vi "main.vi"() -> ()   [LabVIEW 2014]
uses:
  libraryGcode/ControlGlobal/stateModeDevice.ctl
  libraryGcode/control/stateBoardFirmware.ctl
  libraryGcode/control/Queue/QueueCMDandPOS.ctl
  libraryGcode/control/Queue/TypeDataPOS.ctl
  libraryGcode/control/stateCmdUpdatePara.ctl
  C/Users/annha/Desktop/Inverse Kinematic - demo/controls/Robot_definition.ctl
  LIN3D/Robot_testing_instructions.ctl
  libraryGcode/control/TypeFirmwareControl.ctl
  libraryGcode/ClassStringGcode/XuLyDataDisplay.lvclass
  <vilib>/Platform/TimedLoop/XDataNode/timing_clust.ctl
  <vilib>/Platform/TimedLoop/XDataNode/nitl_modes.ctl
  <vilib>/Platform/TimedLoop/XDataNode/wakeup.ctl
  libraryGcode/ClassParameter/stateLoop_View.ctl
  libraryGcode/ClassStringGcode/SelectMcode.ctl
  libraryGcode/ClassStringGcode/SelectGcode.ctl
  libraryGcode/variableGlobal/StartAutoandGcode.vi
  <vilib>/Platform/TimedLoop/XDataNode/XDataNode.xnode
  libraryGcode/LibraryGcode.lvlib
  <vilib>/Platform/TimedLoop/XDataNode/XDNodeRunTimeDep.lvlib
  <vilib>/picture/3D Picture Control/NI_3D Picture Control.lvlib
  libraryGcode/ClassParameter/ParameterConf.lvclass
panel:
  out "degrees":cluster{"A":dbl, "B":dbl}
  out "error out 2":errorcluster
  out "error out":errorcluster
  out "data GET":string="w\n"
  out "POS":cluster{"X":dbl, "Y":dbl, "Z":dbl}
  out "STATE BOARD":T1=enum."Waiting"
  out "statusMode":T2=enum."Menu"
  in  "SwitchMode":bool
  in  "Exit Program":bool=TRUE
  in  "Tab Control":enum32{"Setting", "Auto", "Config", ""}(tab)
  out "G2-G3 PARA":cluster{"X":dbl, "Y":dbl, "I":dbl, "J":dbl}
  in  "Send Gcode manual":T3
  in  "BUTTON CONTROL GCODE FILE":T4={"FILE"={"AddFile_ButtonSaveFile"=FALSE, "AddFile_ButtonDeleteLastLine"=FALSE, "AddFile_ButtonDeleteAll"=FALSE}, "MOTION"={"AddFile_ButtonGoHome"=TRUE, "AddFile_ButtonAddG1"=FALSE, "AddFile_ButtonAddG0"=FALSE}}
  in  "BUTTON CONTROL MANUAL":T5
  in  "PARA":cluster{"STEP":i16, "FEEDRATE":dbl}={"STEP"=10, "FEEDRATE"=500.0} {"FEEDRATE" min=0.0 max=10000.0 step=50.0; "STEP" min=0 max=90 step=2 format="%-1.0f"}
  in  "CONTROL PWM":T6={"SPIN"={"PWM"=55.0, "Control_buttonSpindle"=FALSE, "ButtonSPINDLE_ADD_FILE"=FALSE}, "FAN 1"={"Control_ButtonFan1"=FALSE, "PWM"=255.0, "AddFile_ButtonFan1"=FALSE}, "FAN 2"={"PWM"=0.0, "Control_ButtonFan2"=FALSE, "AddFile_ButtonFan2"=FALSE}, "FAN 3"={"PWM"=0.0, "Control_ButtonFan3"=FALSE, "AddFile_ButtonFan3"=FALSE}, "WAIT PIN"={"PIN INPUT"=55.0, "Control_ButtonWaitPin"=FALSE, "AddFile_ButtonWaitPin"=FALSE}, "SOLENOID"={"Control_ButtonSolenoid"=FALSE, "AddFile_ButtonSolenoid"=FALSE}} {"WAIT PIN"."PIN INPUT" min=55.0 max=58.0 step=1.0; "FAN 3"."PWM" min=0.0 max=255.0 step=5.0; "FAN 2"."PWM" min=0.0 max=255.0 step=5.0; "FAN 1"."PWM" min=0.0 max=255.0 step=10.0; "SPIN"."PWM" min=0.0 max=255.0 step=1.0}
  in  "Link Save File":path
  out "GCODE ADD":string="\r"
  in  "File to Cut":path
  in  "Start Auto":bool
  out "G-Code Array 2":string[](array[string])=["Loi khong ket noChua Chon File"]
  in  "RESET ERROR":bool
  in  "MAX FEEDRATE":T7={"DATA"={"X"=4000.0, "Y"=4000.0, "Z"=4000.0}, "Config_SetFeedrate"=FALSE}
  in  "MAX ACCEL":T8={"DATA"={"X"=5000.0, "Y"=5000.0, "Z"=500.0}, "Config_SetMaxACCEL"=FALSE}
  in  "STEPSIZE":T9={"DATA"={"X"=88.89, "Y"=88.89, "Z"=2133.33}, "Config_SetStepSize"=FALSE}
  in  "M204 Start AcceL":T10={"Config_SetSTARTACCEL"=FALSE, "data"={"P"=88.89, "R"=88.89, "T"=2133.33}}
  in  "Move":cluster{"X":dbl, "Y":dbl, "OK Button":bool}
  in  "Config_SaveEEPROM":bool
  out "output cluster 2":cluster{"angle 1":dbl, "angle 2":dbl, i32}
  out "3D Picture":refnum<vi>(3d-picture)
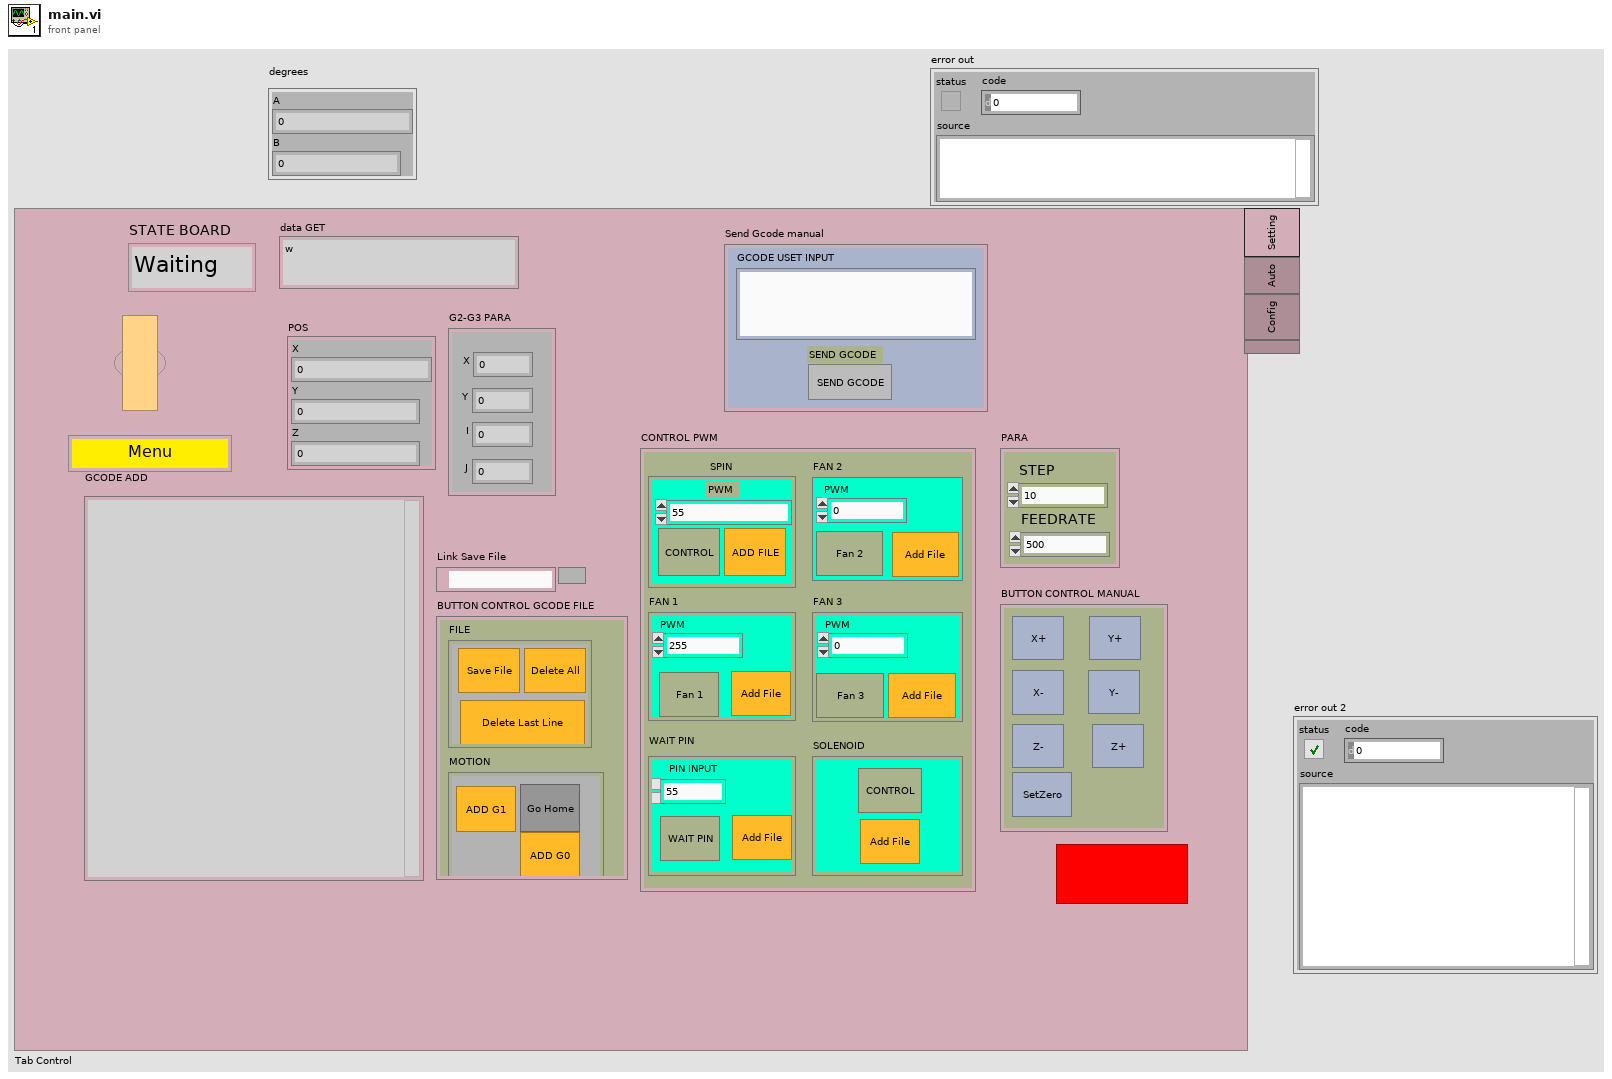
[diagram p1: front panel]
types:
  T1 = typedef "LibraryGcode.lvlib/stateBoardFirmware.ctl" = enum16{"Running", "Waiting", "Pos", "IDLE"}
  T2 = typedef "stateModeDevice.ctl" = enum16{"Auto", "Menu", "WaitAutoFinish", "Config", "initAuto"}
  T3 = cluster{"GCODE USET INPUT":string, "SEND GCODE":bool}
  T4 = cluster{"FILE":cluster{"AddFile_ButtonSaveFile":bool, "AddFile_ButtonDeleteLastLine":bool, "AddFile_ButtonDeleteAll":bool}, "MOTION":cluster{"AddFile_ButtonGoHome":bool, "AddFile_ButtonAddG1":bool, "AddFile_ButtonAddG0":bool}}
  T5 = cluster{"Control_ButtonX+":bool, "Control_ButtonX-":bool, "Control_ButtonY+":bool, "Control_ButtonY-":bool, "Control_ButtonZ+":bool, "Control_ButtonZ-":bool, "Control_ButtonSetZero":bool}
  T6 = cluster{"SPIN":cluster{"PWM":dbl, "Control_buttonSpindle":bool, "ButtonSPINDLE_ADD_FILE":bool}, "FAN 1":cluster{"Control_ButtonFan1":bool, "PWM":dbl, "AddFile_ButtonFan1":bool}, "FAN 2":cluster{"PWM":dbl, "Control_ButtonFan2":bool, "AddFile_ButtonFan2":bool}, "FAN 3":cluster{"PWM":dbl, "Control_ButtonFan3":bool, "AddFile_ButtonFan3":bool}, "WAIT PIN":cluster{"PIN INPUT":dbl, "Control_ButtonWaitPin":bool, "AddFile_ButtonWaitPin":bool}, "SOLENOID":cluster{"Control_ButtonSolenoid":bool, "AddFile_ButtonSolenoid":bool}}
  T7 = cluster{"DATA":cluster{"X":dbl, "Y":dbl, "Z":dbl}, "Config_SetFeedrate":bool}
  T8 = cluster{"DATA":cluster{"X":dbl, "Y":dbl, "Z":dbl}, "Config_SetMaxACCEL":bool}
  T9 = cluster{"DATA":cluster{"X":dbl, "Y":dbl, "Z":dbl}, "Config_SetStepSize":bool}
  T10 = cluster{"Config_SetSTARTACCEL":bool, "data":cluster{"P":dbl, "R":dbl, "T":dbl}}
  T11 = typedef "Robot_testing_instructions.ctl" = enum16{"idle", "Draw Robot", "Init 1 - Application", "Quit", "Close", "Error Handling", "Calculates"}
  T12 = typedef "Robot_definition.ctl" = cluster{"L2":sgl, "L3":sgl, "L1":sgl, "Base":sgl, "X0":sgl, "Z0":sgl}
  T13 = cluster{"Scene ref":refnum<vi>, "Arm 1 ref":refnum<vi>, "Arm 2 ref":refnum<vi>, "Arm 1 offset":cluster{"X":sgl, "Y":sgl, "Z":sgl}[], "Arm 2 offset":cluster{"X":sgl, "Y":sgl, "Z":sgl}[], "sand box":refnum<vi>, "Status":string, "A1":dbl, "A2":dbl, "Robot Definition":T12}
  T14 = typedef "LibraryGcode.lvlib/stateCmdUpdatePara.ctl" = enum16{"updatePos", "UpdateConfigAccel", "UpdateConfigFeed", "UpdateConfigUnit", "UpdateConfigStartAccel", "NoUpdate"}
  T15 = cluster{"Command":T14, "POS":cluster{"X":dbl, "Y":dbl, "Z":dbl}, "DEGREES":cluster{"X":dbl, "Y":dbl}}
  T16 = typedef "LibraryGcode.lvlib/QueueCMDandPOS.ctl" = cluster{"Serial Data Gcode":refnum<queue>, "cmdUpdateDisplay":refnum<queue>}
  T17 = typedef "LibraryGcode.lvlib/TypeFirmwareControl.ctl" = enum16{"ScaraMarlin", "CncMarlin", "Mk4Due"}
  T18 = typedef "XDNodeRunTimeDep.lvlib/timing_clust.ctl" = cluster{"Expected End [f-1]":u64, "Actual End [f-1]":u64, "Finished Late? [f-1]":bool, "Expected End [i-1]":u64, "Actual End [i-1]":u64, "Finished Late? [i-1]":bool, "Expected Start [i]":u64, "Actual Start [i]":u64, "Expected Start [f]":u64, "Actual Start [f]":u64, "Source Name":string, "Structure Name":string, "Period":i64, "Deadline":i64, "Offset":i64, "Start":i64, "Priority":i32, "Timeout":i32, "Mode":T19, "Wakeup Reason":T20, "Error":errorcluster, "Source Type":string, "Secondary Source Type":string, "Global End Time":u64, "Global Start Time":u64, "Frame Duration":u64, "Iteration Duration":u64, "Assigned CPU":i32, "I/O Scan Engine Mode":u32}
  T19 = typedef "XDNodeRunTimeDep.lvlib/nitl_modes.ctl" = enum32{"No Change", "Process missed periods, maintain original phase", "Discard missed periods, maintain original phase", "Process missed periods, ignore original phase", "Discard missed periods, ignore original phase"}
  T20 = typedef "XDNodeRunTimeDep.lvlib/wakeup.ctl" = enum32{"Normal", "Aborted", "Asynchronous wakeup", "Timing source error", "Timed loop error", "Timeout"}
  T21 = typedef "LibraryGcode.lvlib/XuLyDataDisplay.lvclass/SelectMcode.ctl" = enum16{"M204_SetStartingAcceleration", "M503_ReportSetting", "M500_SaveEprom", "M114_GetPosition", "M92_SetAxisStepPerUnit", "M17_EnableStep", "M18_DisableStep", "M80_PowerOn", "M81_PowerOff", "M112_EMGStop", "M118_SerialPrint", "M226_WaitforPinState", "M400_WaitFinishMove", "M203_SetMaxFeedRate", "M201_SetMaxACCEL", "M380_381_SetSoleNoid_On_Off", "M42_InitPin", "M42_PinControl", "M106_SetFan1", "M106_SetFan2", "M106_SetFan3", "M3_SetSpindle", "M5_OffSpindle", "M999_RestartStop"}
  T22 = typedef "LibraryGcode.lvlib/ParameterConf.lvclass/stateLoop_View.ctl" = enum16{"Running", "writeGlobal", "schedules500ms", "init", "End"}
  T23 = enum16{"Fan1", "Fan2", "Fan3", "PARA", "POS_DEGREE", "Solenoid", "Spindle", "TypeFirmware", "WaitPin", "MaxAcel", "MaxFeedrate", "MaxSize", "MaxStartAccel"}
  T24 = typedef "LibraryGcode.lvlib/XuLyDataDisplay.lvclass/SelectGcode.ctl" = enum16{"G0LinearMove", "G1XY", "G1LinearMove", "G2Arc", "G4Dwell", "G20InchUnit", "G21MilliUnit", "G28AutoHome", "G92SetPosition", "G90", "G91RelativePos", "JogX+", "JogX-", "JogY+", "JogY-", "JogZ+", "JogZ-", "sendGcodeString"}
  T25 = cluster{"SPIN":dbl, "FAN2":dbl, "FAN1":dbl, "FAN3":dbl, "WAIT PIN ":dbl}
  T26 = cluster{"PWM":dbl, "TypeFirmware":T17, "XYZ":cluster{"X":dbl, "Y":dbl, "Z":dbl}, "PARA":cluster{"STEP":i16, "FEEDRATE":dbl}, "DEGREES":cluster{"X":dbl, "Y":dbl}, "Solenoid":bool, "StartAccel":cluster{"P":dbl, "R":dbl, "T":dbl}}
  T27 = typedef "Robot_creation_loop_data.ctl" = cluster{"Robot Definition":T12, "Dispenser ref":refnum<vi>, "Arm 2 ref":refnum<vi>, "Arm 1 ref":refnum<vi>, "Base ref":refnum<vi>, "Scene ref":refnum<vi>, "Sand box ref":refnum<vi>, "Arm 1 Offset":cluster{"X":sgl, "Y":sgl, "Z":sgl}[], "Arm 2 Offset":cluster{"X":sgl, "Y":sgl, "Z":sgl}[], "Width":sgl}
  T28 = cluster{"error out":errorcluster, "error IO 2":errorcluster}
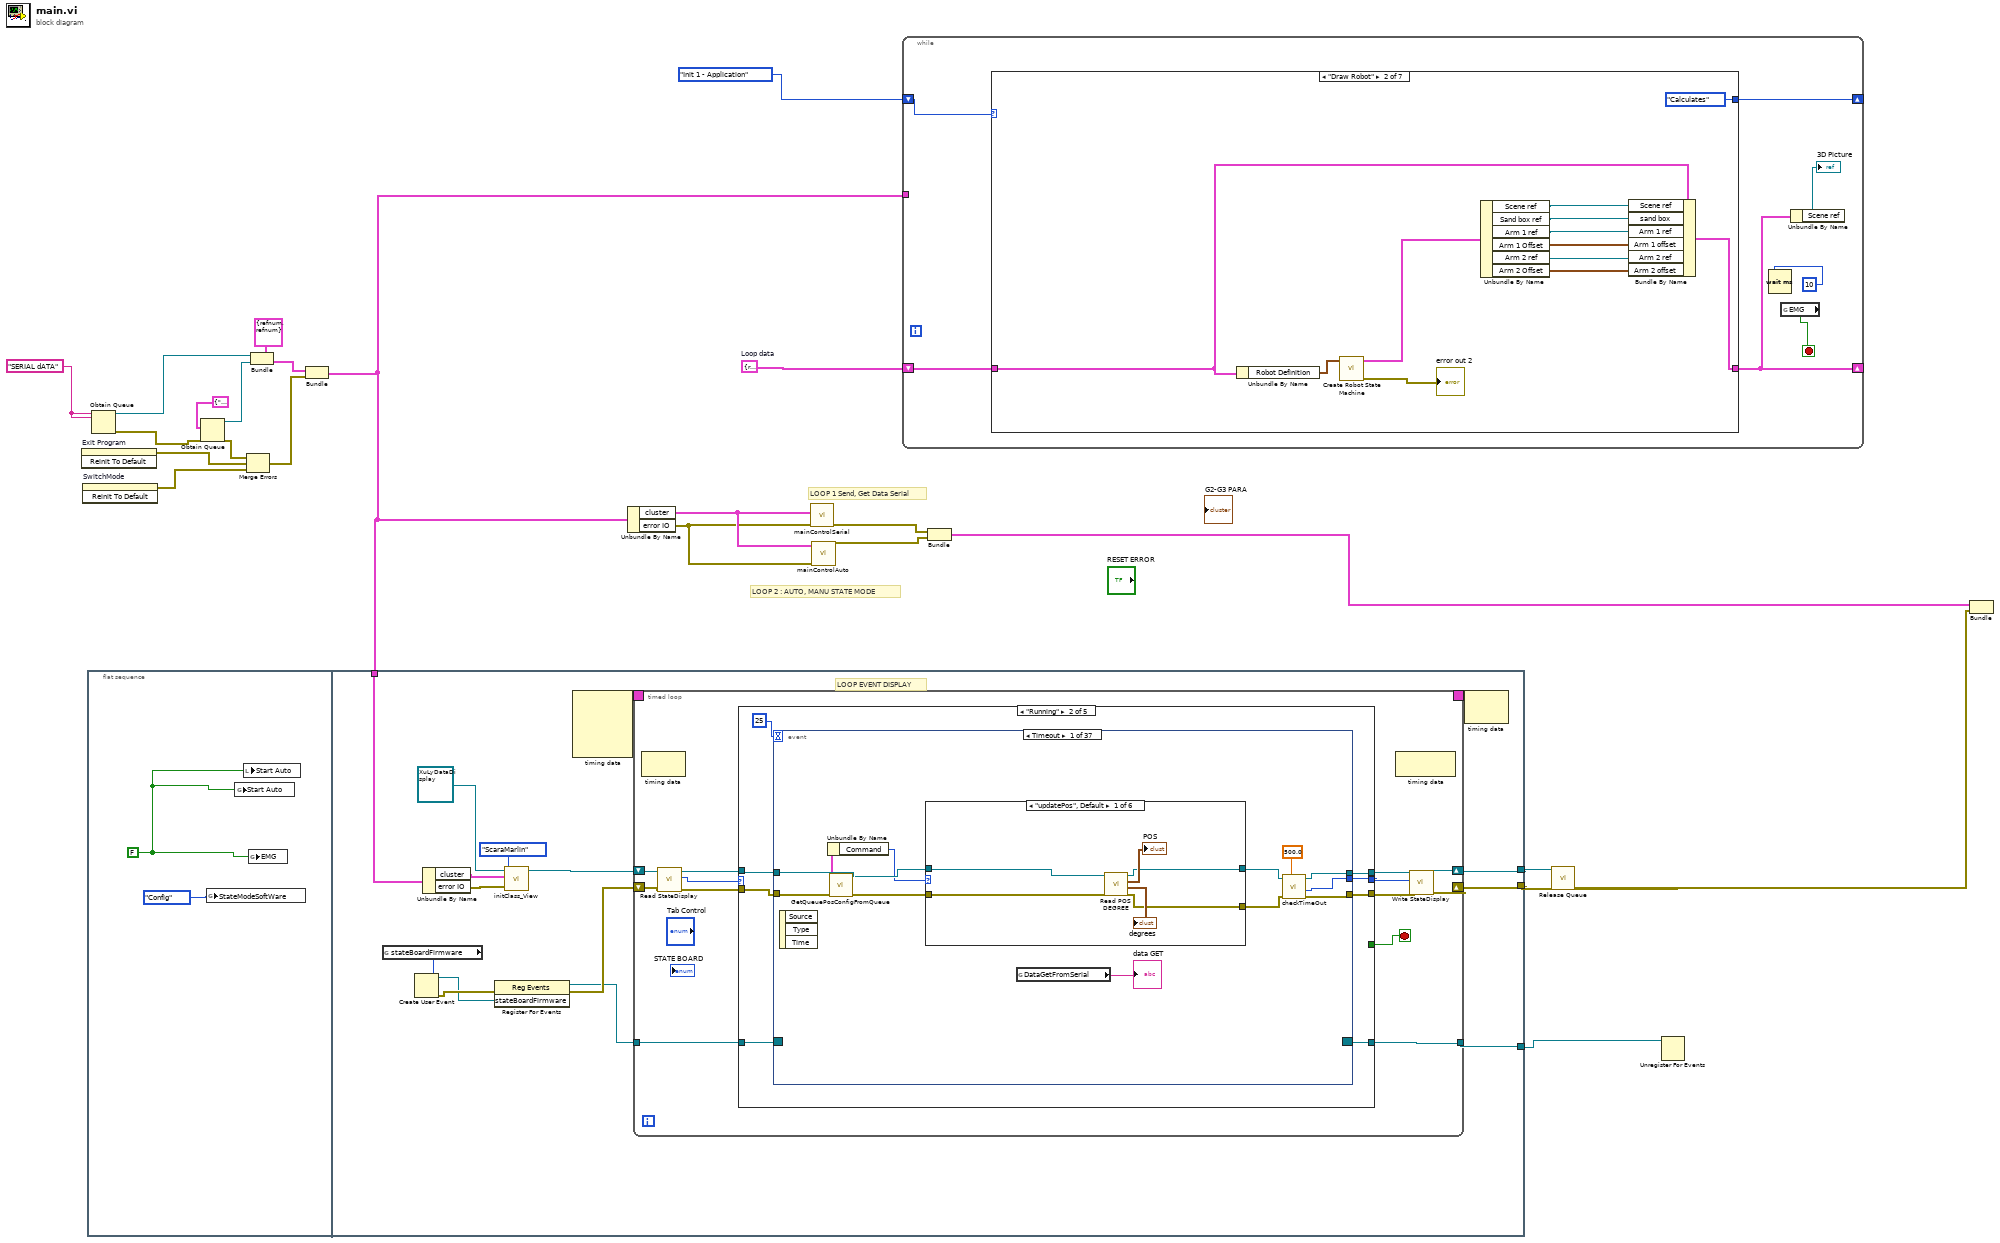
[diagram p0: block diagram]
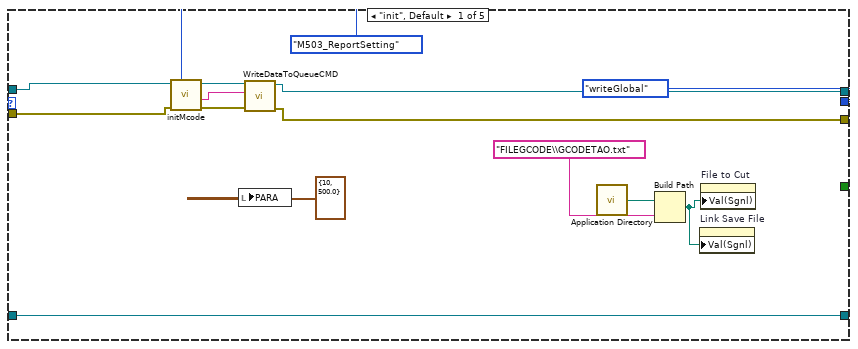
[diagram p2: hidden frame]
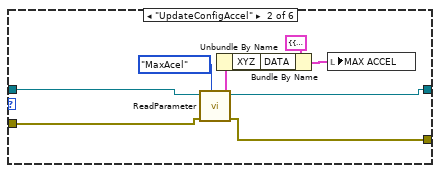
[diagram p3: hidden frame]
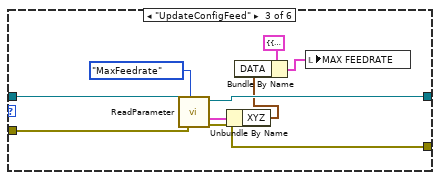
[diagram p4: hidden frame]
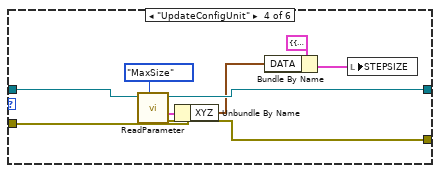
[diagram p5: hidden frame]
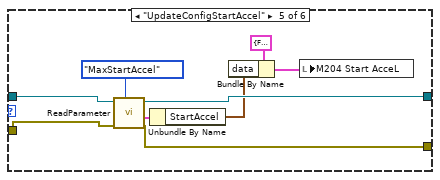
[diagram p6: hidden frame]
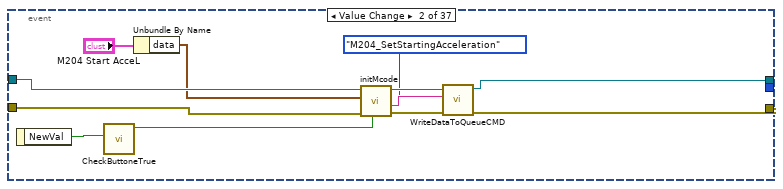
[diagram p8: hidden frame]
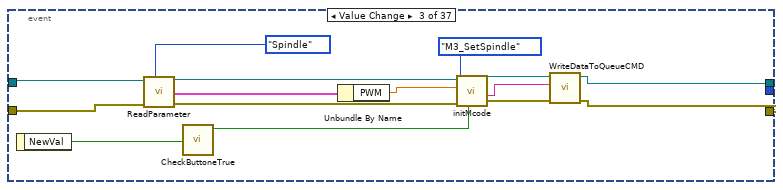
[diagram p9: hidden frame]
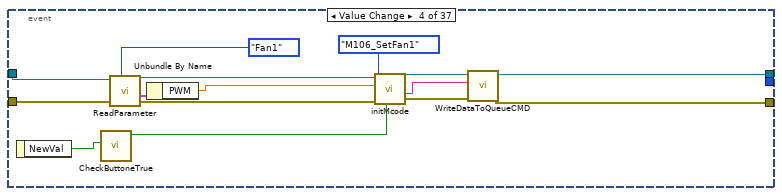
[diagram p10: hidden frame]
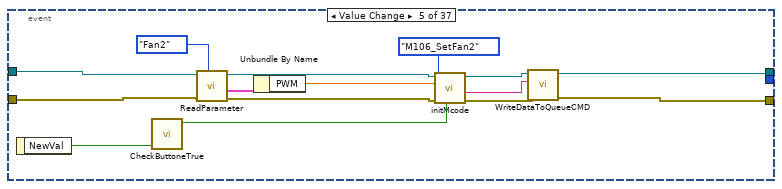
[diagram p11: hidden frame]
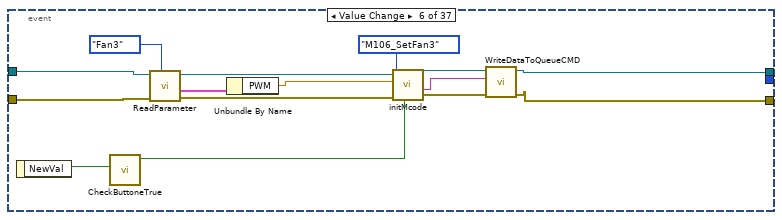
[diagram p12: hidden frame]
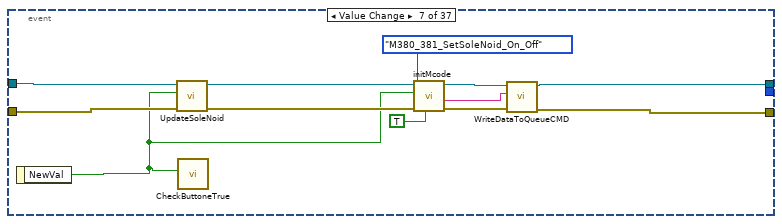
[diagram p13: hidden frame]
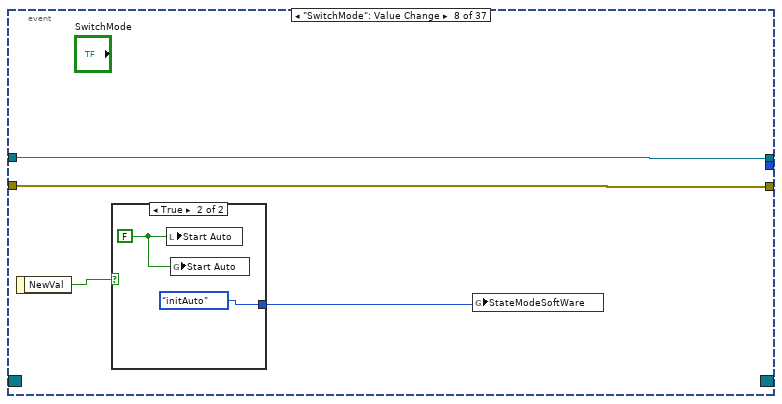
[diagram p14: hidden frame]
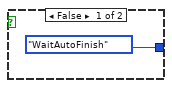
[diagram p15: hidden frame]
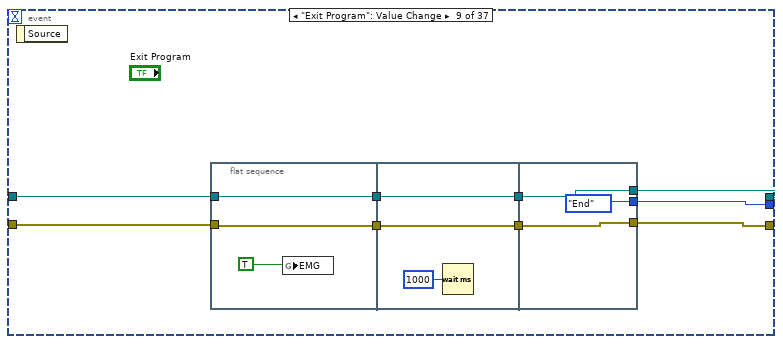
[diagram p16: hidden frame]
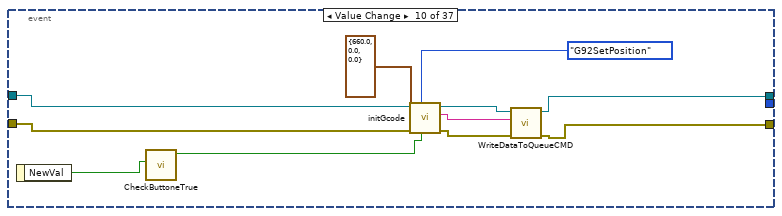
[diagram p17: hidden frame]
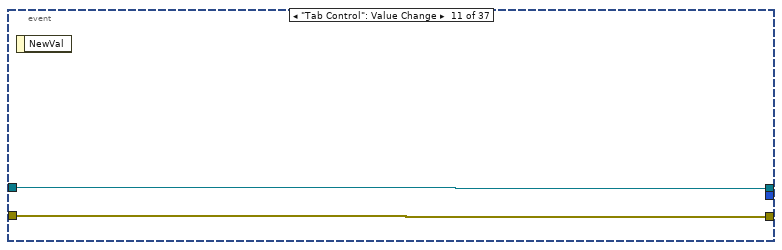
[diagram p18: hidden frame]
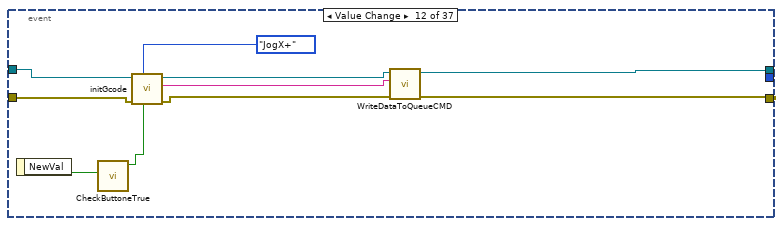
[diagram p19: hidden frame]
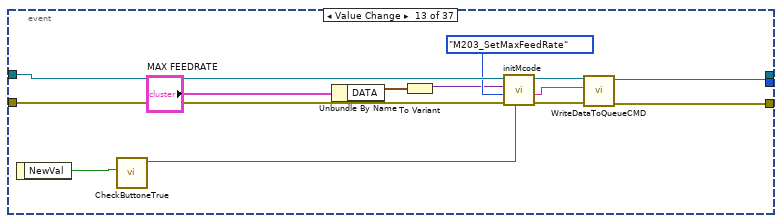
[diagram p20: hidden frame]
diagram:
  w9 = T13 {"Scene ref"=refnum, "Arm 1 ref"=refnum, "Arm 2 ref"=refnum, "Arm 1 offset"=[], "Arm 2 offset"=[], "sand box"=refnum, "Status"="", "A1"=43.0, "A2"=23.0, "Robot Definition"={"L2"=0.0, "L3"=0.0, "L1"=0.0, "Base"=0.0, "X0"=0.0, "Z0"=0.0}}  # Loop data
  w23 = "SERIAL dATA" ("name (unnamed)")
  # "LOOP 2 : AUTO, MANU STATE MODE"
  # "LOOP 1 Send, Get Data Serial"
  n1 = invoke on="Exit Program" class="Bool" method="Reinit To Default"() -> (error out=w21:errorcluster)  [unwired: 3 in, 2 out]
  n2 = invoke on="SwitchMode" class="Bool (strict)" method="Reinit To Default"() -> (error out=w22:errorcluster)  [unwired: 3 in, 2 out]
  n3 = flat-sequence {
    tunnel: [w41] -> w3
    tunnel: w11 -> [w40]
    tunnel: [w37] -> w4
    tunnel: [w27] -> w1
    frame #0 {
      w25 = FALSE ("Start Auto")
      n4 = global write "StartAutoandGcode.vi" "StateModeSoftWare"(stateModeDevice."Config" ("Enum")) -> ()
      n5 = global write "StartAutoandGcode.vi" "Start Auto"(w25) -> ()
      n6 = local write "Start Auto"(w25) -> ()
      n7 = global write "StartAutoandGcode.vi" "EMG"(w25) -> ()
    }
    frame #1 {
      # "LOOP EVENT DISPLAY"
      n8 = global read "StartAutoandGcode.vi" "stateBoardFirmware"() -> (w29:T1)
      n9 = Create User Event(user event datatype=w29) -> (user event=w28:refnum<user-event>, error out=w31:errorcluster)  [unwired: 1 in]
      n10 = Unbundle By Name(w40) -> ("cluster"=w36:T16, "error IO"=w26:errorcluster)
      n11 = register-events(error in=w31, w28) -> (reference out=w30:refnum<event-registration>, error out=w32:errorcluster)  [unwired: 1 in]
      n12 = call-dynamic "initClass_View.vi"("error in (no error)"=w26, "TypeFirmware"=TypeFirmwareControl."ScaraMarlin", "Queue Process"=w36, "XuLyDataDisplay in"=refnum<class "XuLyDataDisplay.lvclass"> refnum) -> ("XuLyDataDisplay out"=w34:refnum<class "XuLyDataDisplay.lvclass">)  [unwired: 6 in, 1 out]
      n13 = node-c288() -> (w39:T18)  [unwired: 4 in]
      n14 = timed-loop {
        timing: w39 -> [_]
        timing-out: [_] -> w38
        shift-right: [w49] -> w37
        shift-left: w34 -> [w53]
        shift-right: [w48] -> w41
        shift-left: w32 -> [w51]
        tunnel: w30 -> [w43]
        tunnel: [w42] -> w27
        stop <- w54 stop-if-true
        n15 = node-c288() -> ()  [unwired: 1 in, 1 out]
        n16 = call-dynamic "Read StateDisplay.vi"("error in (no error)"=w51, "ParameterConf in"=w53) -> ("error out"=w50:errorcluster, "StateDisplay"=w46:T22, "ParameterConf out"=w52:refnum<class "XuLyDataDisplay.lvclass">)  [unwired: 7 in]
        n17 = case shown="\"Running\"" w46 {
          tunnel: w50 -> [w61 w71 w542 w554 w571]
          tunnel: [_ _ TRUE _ _] -> w54
          tunnel: [w60 w75 w542 w552 w568] -> w47
          tunnel: w52 -> [w65 w77 w541 w555 w572]
          tunnel: [w62 w73 w541 w553 w569] -> w44
          tunnel: [stateLoop_View."writeGlobal" ("StateDisplay") w76 stateLoop_View."init" ("StateDisplay") stateLoop_View."schedules500ms" ("StateDisplay") stateLoop_View."Running" ("StateDisplay")] -> w45
          tunnel: w43 -> [w57 w74 w539 w544 w566]
          tunnel: [w57 w72 w539 w544 w566] -> w42
          frame "init", Default {
            n18 = call-dynamic "initMcode.vi"("error in (no error)"=w61, "mCode"=SelectMcode."M503_ReportSetting", "XuLyDataDisplay in"=w65) -> ("error out"=w59:errorcluster, "McodeOut"=w63:string, "XuLyDataDisplay out"=w64:refnum<class "XuLyDataDisplay.lvclass">)  [unwired: 6 in]
            n19 = local write "PARA"(cluster{"STEP":i16, "FEEDRATE":dbl} {"STEP"=10, "FEEDRATE"=500.0} ("PARA")) -> ()
            n20 = call-dynamic "WriteDataToQueueCMD.vi"("error in (no error)"=w59, "DataIn"=w63, "ParameterConf in"=w64) -> ("error out"=w60:errorcluster, "ParameterConf out"=w62:refnum<class "XuLyDataDisplay.lvclass">)  [unwired: 7 in]
            n21 = call <vilib>:"Application Directory.vi"() -> ("Application Directory"=w68:path)
            n22 = Build Path(base path=w68, name or relative path="FILEGCODE\\GCODETAO.txt") -> (appended path=w70:path)
            n23 = property on="Link Save File" class="Path"("Val(Sgnl)"=w70) -> ()  [unwired: 2 in, 2 out]
            n24 = property on="File to Cut" class="Path"("Val(Sgnl)"=w70) -> ()  [unwired: 2 in, 2 out]
          }
          frame "Running" {
            n25 = event shown="[0] Timeout" {
              selector: w74 -> [_ _ _ _ _ _ _ _ _ _ _ _ _ _ _ _ _ _ _ _ _ _ _ _ _ _ _ _ _ _ _ _ _ w498 _ _ _]
              dyn-events: [_ _ _ _ _ _ _ _ _ _ _ _ _ _ _ _ _ _ _ _ _ _ _ _ _ _ _ _ _ _ _ _ _ w498 _ _ _] -> w72
              timeout: 25 -> [_ _ _ _ _ _ _ _ _ _ _ _ _ _ _ _ _ _ _ _ _ _ _ _ _ _ _ _ _ _ _ _ _ _ _ _ _]
              tunnel: w71 -> [w90 w140 w160 w175 w190 w206 w218 w223 w229 w252 w257 w262 w274 w290 w299 w313 w326 w332 w344 w357 w363 w382 w397 w408 w425 w440 w446 w450 w452 w461 w473 w483 w495 w506 w516 w522 w532]
              tunnel: [w82 w143 w151 w171 w184 w200 w212 w223 w228 w247 w257 w260 w276 w285 w301 w310 w321 w332 w336 w357 w362 w369 w385 w400 w415 w428 w443 w450 w453 w464 w467 w484 w493 w502 w509 w519 w531] -> w75
              tunnel: w77 -> [w91 w146 w161 w176 w191 w205 w219 w222 w232 w253 w256 w263 w278 w291 w304 w314 w328 w331 w345 w358 w364 w383 w398 w409 w426 w441 w447 w449 w455 w463 w474 w486 w496 w507 w517 w523 w533]
              tunnel: [w83 w144 w152 w172 w185 w201 w215 w222 w235 w248 w256 w258 w275 w286 w302 w311 w319 w331 w335 w358 w359 w370 w386 w401 w416 w429 w444 w449 w451 w456 w468 w485 w494 w503 w510 w520 w529] -> w73
              tunnel: [w80 _ _ _ _ _ _ _ w227 _ _ _ _ _ _ _ _ _ _ stateLoop_View."writeGlobal" ("StateDisplay") _ _ _ _ _ _ _ _ _ _ _ _ _ _ _ _ _] -> w76
              event Timeout {
                n26 = event-data() -> ()  [unwired: 1 in, 3 out]
                n27 = call-dynamic "GetQueuePosConfigFromQueue.vi"("error in (no error)"=w90, "ParameterConf in"=w91) -> ("error out"=w87:errorcluster, "element"=w89:T15, "ParameterConf out"=w88:refnum<class "XuLyDataDisplay.lvclass">)  [unwired: 7 in]
                n28 = Unbundle By Name(w89) -> ("Command"=w79:T14)
                n29 = case shown="\"updatePos\", Default" w79 {
                  tunnel: [w93 w106 w113 w123 w132 w135] -> w85
                  tunnel: w88 -> [w95 w105 w115 w116 w128 w135]
                  tunnel: [w92 w103 w112 w122 w131 w134] -> w84
                  tunnel: w87 -> [w94 w104 w114 w124 w133 w134]
                  frame "updatePos", Default {
                    n30 = call-dynamic "Read POS DEGREE.vi"("error in (no error)"=w94, "ParameterConf in"=w95) -> ("error out"=w92:errorcluster, "DEGREES"=→"degrees":cluster{"X":dbl, "Y":dbl}, "POS"=→"POS":cluster{"X":dbl, "Y":dbl, "Z":dbl}, "ParameterConf out"=w93:refnum<class "XuLyDataDisplay.lvclass">)  [unwired: 6 in]
                  }
                  frame "UpdateConfigAccel" {
                    n31 = call-dynamic "ReadParameter.vi"("ParameterConf in"=w105, "error in (no error)"=w104, "Parameter"=T23."MaxAcel") -> ("ParameterConf out"=w106:refnum<class "XuLyDataDisplay.lvclass">, "DataOutClust"=w99:T26, "error out"=w103:errorcluster)  [unwired: 4 in, 1 out]
                    n32 = Unbundle By Name(w99) -> ("XYZ"=w98:cluster{"X":dbl, "Y":dbl, "Z":dbl})
                    n33 = Bundle By Name(cluster=T8 {"DATA"={"X"=355.0, "Y"=355.0, "Z"=2133.0}, "Config_SetMaxACCEL"=FALSE} ("MAX ACCEL"), "DATA"=w98) -> (w101:T8)
                    n34 = local write "MAX ACCEL"(w101) -> ()
                  }
                  frame "UpdateConfigFeed" {
                    n35 = call-dynamic "ReadParameter.vi"("ParameterConf in"=w115, "error in (no error)"=w114, "Parameter"=T23."MaxFeedrate") -> ("ParameterConf out"=w113:refnum<class "XuLyDataDisplay.lvclass">, "DataOutClust"=w108:T26, "error out"=w112:errorcluster)  [unwired: 4 in, 1 out]
                    n36 = Unbundle By Name(w108) -> ("XYZ"=w107:cluster{"X":dbl, "Y":dbl, "Z":dbl})
                    n37 = Bundle By Name(cluster=T9 {"DATA"={"X"=355.56, "Y"=355.56, "Z"=2133.33}, "Config_SetStepSize"=FALSE} ("STEPSIZE"), "DATA"=w107) -> (w110:T9)
                    n38 = local write "MAX FEEDRATE"(w110) -> ()
                  }
                  frame "UpdateConfigUnit" {
                    n39 = call-dynamic "ReadParameter.vi"("ParameterConf in"=w116, "error in (no error)"=w124, "Parameter"=T23."MaxSize") -> ("ParameterConf out"=w123:refnum<class "XuLyDataDisplay.lvclass">, "DataOutClust"=w118:T26, "error out"=w122:errorcluster)  [unwired: 4 in, 1 out]
                    n40 = Unbundle By Name(w118) -> ("XYZ"=w117:cluster{"X":dbl, "Y":dbl, "Z":dbl})
                    n41 = Bundle By Name(cluster=T7 {"DATA"={"X"=150000.0, "Y"=150000.0, "Z"=10000.0}, "Config_SetFeedrate"=FALSE} ("MAX FEEDRATE"), "DATA"=w117) -> (w120:T7)
                    n42 = local write "STEPSIZE"(w120) -> ()
                  }
                  frame "UpdateConfigStartAccel" {
                    n43 = call-dynamic "ReadParameter.vi"("ParameterConf in"=w128, "error in (no error)"=w133, "Parameter"=T23."MaxStartAccel") -> ("ParameterConf out"=w132:refnum<class "XuLyDataDisplay.lvclass">, "DataOutClust"=w126:T26, "error out"=w131:errorcluster)  [unwired: 4 in, 1 out]
                    n44 = Unbundle By Name(w126) -> ("StartAccel"=w125:cluster{"P":dbl, "R":dbl, "T":dbl})
                    n45 = Bundle By Name(cluster=T10 {"Config_SetSTARTACCEL"=FALSE, "data"={"P"=355.56, "R"=355.56, "T"=2133.33}} ("M204 Start AcceL"), "data"=w125) -> (w129:T10)
                    n46 = local write "M204 Start AcceL"(w129) -> ()
                  }
                  frame "NoUpdate" {
                  }
                }
                n47 = global read "StartAutoandGcode.vi" "DataGetFromSerial"() -> (→"data GET":string)
                n48 = call-dynamic "checkTimeOut.vi"("error in (no error)"=w84, "Time"=500.0, "ParameterConf in"=w85) -> ("error out"=w82:errorcluster, "stateDisplay"=w80:T22, "ParameterConf out"=w83:refnum<class "XuLyDataDisplay.lvclass">)  [unwired: 5 in, 1 out]
              }
              event "M204 Start AcceL.Config_SetSTARTACCEL": Value Change {
                n49 = event-data() -> ("NewVal"=w147:bool)  [unwired: 1 in]
                n50 = call "CheckButtoneTrue.vi"("IN"=w147) -> ("OUT"=w136:bool)  [unwired: 10 in]
                n51 = Unbundle By Name("M204 Start AcceL") -> ("data"=w138:cluster{"P":dbl, "R":dbl, "T":dbl})
                n52 = call-dynamic "initMcode.vi"("CheckMenu"=w136, "error in (no error)"=w140, "mCode"=SelectMcode."M204_SetStartingAcceleration", "DataVariant"=w138, "XuLyDataDisplay in"=w146) -> ("error out"=w142:errorcluster, "McodeOut"=w141:string, "XuLyDataDisplay out"=w145:refnum<class "XuLyDataDisplay.lvclass">)  [unwired: 4 in]
                n53 = call-dynamic "WriteDataToQueueCMD.vi"("error in (no error)"=w142, "DataIn"=w141, "ParameterConf in"=w145) -> ("error out"=w143:errorcluster, "ParameterConf out"=w144:refnum<class "XuLyDataDisplay.lvclass">)  [unwired: 7 in]
              }
              event "CONTROL PWM.SPIN.Control_buttonSpindle": Value Change {
                n54 = event-data() -> ("NewVal"=w162:bool)  [unwired: 1 in]
                n55 = call-dynamic "ReadParameter.vi"("ParameterConf in"=w161, "error in (no error)"=w160, "Parameter"=T23."Spindle") -> ("ParameterConf out"=w158:refnum<class "XuLyDataDisplay.lvclass">, "DataOutClust"=w150:T26, "error out"=w157:errorcluster)  [unwired: 4 in, 1 out]
                n56 = call "CheckButtoneTrue.vi"("IN"=w162) -> ("OUT"=w155:bool)  [unwired: 10 in]
                n57 = Unbundle By Name(w150) -> ("PWM"=w149:dbl)
                n58 = call-dynamic "initMcode.vi"("CheckMenu"=w155, "error in (no error)"=w157, "mCode"=SelectMcode."M3_SetSpindle", "DataVariant"=w149, "XuLyDataDisplay in"=w158) -> ("error out"=w156:errorcluster, "McodeOut"=w154:string, "XuLyDataDisplay out"=w159:refnum<class "XuLyDataDisplay.lvclass">)  [unwired: 4 in]
                n59 = call-dynamic "WriteDataToQueueCMD.vi"("error in (no error)"=w156, "DataIn"=w154, "ParameterConf in"=w159) -> ("error out"=w151:errorcluster, "ParameterConf out"=w152:refnum<class "XuLyDataDisplay.lvclass">)  [unwired: 7 in]
              }
              event "CONTROL PWM.FAN 1.Control_ButtonFan1": Value Change {
                n60 = event-data() -> ("NewVal"=w177:bool)  [unwired: 1 in]
                n61 = call "CheckButtoneTrue.vi"("IN"=w177) -> ("OUT"=w166:bool)  [unwired: 10 in]
                n62 = call-dynamic "ReadParameter.vi"("ParameterConf in"=w176, "error in (no error)"=w175, "Parameter"=T23."Fan1") -> ("ParameterConf out"=w174:refnum<class "XuLyDataDisplay.lvclass">, "DataOutClust"=w165:T26, "error out"=w170:errorcluster)  [unwired: 4 in, 1 out]
                n63 = Unbundle By Name(w165) -> ("PWM"=w164:dbl)
                n64 = call-dynamic "initMcode.vi"("CheckMenu"=w166, "error in (no error)"=w170, "mCode"=SelectMcode."M106_SetFan1", "DataVariant"=w164, "XuLyDataDisplay in"=w174) -> ("error out"=w168:errorcluster, "McodeOut"=w167:string, "XuLyDataDisplay out"=w173:refnum<class "XuLyDataDisplay.lvclass">)  [unwired: 4 in]
                n65 = call-dynamic "WriteDataToQueueCMD.vi"("error in (no error)"=w168, "DataIn"=w167, "ParameterConf in"=w173) -> ("error out"=w171:errorcluster, "ParameterConf out"=w172:refnum<class "XuLyDataDisplay.lvclass">)  [unwired: 7 in]
              }
              event "CONTROL PWM.FAN 2.Control_ButtonFan2": Value Change {
                n66 = event-data() -> ("NewVal"=w192:bool)  [unwired: 1 in]
                n67 = call "CheckButtoneTrue.vi"("IN"=w192) -> ("OUT"=w182:bool)  [unwired: 10 in]
                n68 = call-dynamic "ReadParameter.vi"("ParameterConf in"=w191, "error in (no error)"=w190, "Parameter"=T23."Fan2") -> ("ParameterConf out"=w189:refnum<class "XuLyDataDisplay.lvclass">, "DataOutClust"=w180:T26, "error out"=w183:errorcluster)  [unwired: 4 in, 1 out]
                n69 = Unbundle By Name(w180) -> ("PWM"=w178:dbl)
                n70 = call-dynamic "initMcode.vi"("CheckMenu"=w182, "error in (no error)"=w183, "mCode"=SelectMcode."M106_SetFan2", "DataVariant"=w178, "XuLyDataDisplay in"=w189) -> ("error out"=w186:errorcluster, "McodeOut"=w188:string, "XuLyDataDisplay out"=w187:refnum<class "XuLyDataDisplay.lvclass">)  [unwired: 4 in]
                n71 = call-dynamic "WriteDataToQueueCMD.vi"("error in (no error)"=w186, "DataIn"=w188, "ParameterConf in"=w187) -> ("error out"=w184:errorcluster, "ParameterConf out"=w185:refnum<class "XuLyDataDisplay.lvclass">)  [unwired: 7 in]
              }
              event "CONTROL PWM.FAN 3.Control_ButtonFan3": Value Change {
                n72 = event-data() -> ("NewVal"=w207:bool)  [unwired: 1 in]
                n73 = call "CheckButtoneTrue.vi"("IN"=w207) -> ("OUT"=w196:bool)  [unwired: 10 in]
                n74 = call-dynamic "ReadParameter.vi"("ParameterConf in"=w205, "error in (no error)"=w206, "Parameter"=T23."Fan3") -> ("ParameterConf out"=w204:refnum<class "XuLyDataDisplay.lvclass">, "DataOutClust"=w194:T26, "error out"=w198:errorcluster)  [unwired: 4 in, 1 out]
                n75 = Unbundle By Name(w194) -> ("PWM"=w193:dbl)
                n76 = call-dynamic "initMcode.vi"("CheckMenu"=w196, "error in (no error)"=w198, "mCode"=SelectMcode."M106_SetFan3", "DataVariant"=w193, "XuLyDataDisplay in"=w204) -> ("error out"=w199:errorcluster, "McodeOut"=w203:string, "XuLyDataDisplay out"=w202:refnum<class "XuLyDataDisplay.lvclass">)  [unwired: 4 in]
                n77 = call-dynamic "WriteDataToQueueCMD.vi"("error in (no error)"=w199, "DataIn"=w203, "ParameterConf in"=w202) -> ("error out"=w200:errorcluster, "ParameterConf out"=w201:refnum<class "XuLyDataDisplay.lvclass">)  [unwired: 7 in]
              }
              event "CONTROL PWM.SOLENOID.Control_ButtonSolenoid": Value Change {
                n78 = event-data() -> ("NewVal"=w209:bool)  [unwired: 1 in]
                n79 = call-dynamic "UpdateSoleNoid.vi"("error in (no error)"=w218, "Boolean"=w209, "ParameterConf in"=w219) -> ("error out"=w214:errorcluster, "ParameterConf out"=w217:refnum<class "XuLyDataDisplay.lvclass">)  [unwired: 7 in]
                n80 = call "CheckButtoneTrue.vi"("IN"=w209) -> ()  [unwired: 10 in, 1 out]
                n81 = call-dynamic "initMcode.vi"("CheckMenu"=TRUE, "error in (no error)"=w214, "mCode"=SelectMcode."M380_381_SetSoleNoid_On_Off", "DataVariant"=w209, "XuLyDataDisplay in"=w217) -> ("error out"=w213:errorcluster, "McodeOut"=w210:string, "XuLyDataDisplay out"=w216:refnum<class "XuLyDataDisplay.lvclass">)  [unwired: 4 in]
                n82 = call-dynamic "WriteDataToQueueCMD.vi"("error in (no error)"=w213, "DataIn"=w210, "ParameterConf in"=w216) -> ("error out"=w212:errorcluster, "ParameterConf out"=w215:refnum<class "XuLyDataDisplay.lvclass">)  [unwired: 7 in]
              }
              event "SwitchMode": Value Change {
                n83 = event-data() -> ("NewVal"=w221:bool)  [unwired: 1 in]
                n84 = case shown="True" w221 {
                  tunnel: [stateModeDevice."WaitAutoFinish" ("Enum") stateModeDevice."initAuto" ("Enum")] -> w220
                  frame False {
                  }
                  frame True {
                    w225 = FALSE ("Start Auto")
                    n85 = local write "Start Auto"(w225) -> ()
                    n86 = global write "StartAutoandGcode.vi" "Start Auto"(w225) -> ()
                  }
                }
                n87 = global write "StartAutoandGcode.vi" "StateModeSoftWare"(w220) -> ()
              }
              event "Exit Program": Value Change {
                n88 = event-data() -> ()  [unwired: 1 in, 1 out]
                n89 = flat-sequence {
                  tunnel: [w238] -> w233
                  tunnel: w232 -> [w238]
                  tunnel: [w237] -> w230
                  tunnel: w229 -> [w237]
                  tunnel: [w240] -> w234
                  tunnel: w233 -> [w240]
                  tunnel: [w239] -> w231
                  tunnel: w230 -> [w239]
                  tunnel: [w244] -> w235
                  tunnel: w234 -> [w244]
                  tunnel: [w243] -> w228
                  tunnel: w231 -> [w243]
                  tunnel: [stateLoop_View."End" ("StateDisplay")] -> w227
                  frame #0 {
                    n90 = global write "StartAutoandGcode.vi" "EMG"(TRUE ("EMG1")) -> ()
                  }
                  frame #1 {
                    n91 = Wait (ms)(milliseconds to wait=u32 1000) -> ()  [unwired: 1 out]
                  }
                  frame #2 {
                  }
                }
              }
              event "BUTTON CONTROL MANUAL.Control_ButtonSetZero": Value Change {
                n92 = event-data() -> ("NewVal"=w246:bool)  [unwired: 1 in]
                n93 = call "CheckButtoneTrue.vi"("IN"=w246) -> ("OUT"=w245:bool)  [unwired: 10 in]
                n94 = call-dynamic "initGcode.vi"("Che Do"=w245, "gCode"=SelectGcode."G92SetPosition", "error in (no error)"=w252, "PosSetG92"=cluster{"X":dbl, "Y":dbl, "Z":dbl} {"X"=660.0, "Y"=0.0, "Z"=0.0}, "XuLyDataDisplay in"=w253) -> ("error out"=w249:errorcluster, "GcodeString Out"=w250:string, "XuLyDataDisplay out"=w251:refnum<class "XuLyDataDisplay.lvclass">)  [unwired: 4 in]
                n95 = call-dynamic "WriteDataToQueueCMD.vi"("error in (no error)"=w249, "DataIn"=w250, "ParameterConf in"=w251) -> ("error out"=w247:errorcluster, "ParameterConf out"=w248:refnum<class "XuLyDataDisplay.lvclass">)  [unwired: 7 in]
              }
              event "Tab Control": Value Change {
                n96 = event-data() -> ()  [unwired: 1 in, 1 out]
              }
              event "BUTTON CONTROL MANUAL.Control_ButtonX+": Value Change {
                n97 = event-data() -> ("NewVal"=w267:bool)  [unwired: 1 in]
                n98 = call "CheckButtoneTrue.vi"("IN"=w267) -> ("OUT"=w261:bool)  [unwired: 10 in]
                n99 = call-dynamic "initGcode.vi"("Che Do"=w261, "gCode"=SelectGcode."JogX+", "error in (no error)"=w262, "XuLyDataDisplay in"=w263) -> ("error out"=w265:errorcluster, "GcodeString Out"=w259:string, "XuLyDataDisplay out"=w266:refnum<class "XuLyDataDisplay.lvclass">)  [unwired: 5 in]
                n100 = call-dynamic "WriteDataToQueueCMD.vi"("error in (no error)"=w265, "DataIn"=w259, "ParameterConf in"=w266) -> ("error out"=w260:errorcluster, "ParameterConf out"=w258:refnum<class "XuLyDataDisplay.lvclass">)  [unwired: 7 in]
              }
              event "MAX FEEDRATE.Config_SetFeedrate": Value Change {
                n101 = event-data() -> ("NewVal"=w280:bool)  [unwired: 1 in]
                n102 = call "CheckButtoneTrue.vi"("IN"=w280) -> ("OUT"=w277:bool)  [unwired: 10 in]
                n103 = Unbundle By Name("MAX FEEDRATE") -> ("DATA"=w268:cluster{"X":dbl, "Y":dbl, "Z":dbl})
                n104 = To Variant(anything=w268) -> (Variant=w271:variant)
                n105 = call-dynamic "initMcode.vi"("CheckMenu"=w277, "error in (no error)"=w274, "mCode"=SelectMcode."M203_SetMaxFeedRate", "DataVariant"=w271, "XuLyDataDisplay in"=w278) -> ("error out"=w273:errorcluster, "McodeOut"=w270:string, "XuLyDataDisplay out"=w279:refnum<class "XuLyDataDisplay.lvclass">)  [unwired: 4 in]
                n106 = call-dynamic "WriteDataToQueueCMD.vi"("error in (no error)"=w273, "DataIn"=w270, "ParameterConf in"=w279) -> ("error out"=w276:errorcluster, "ParameterConf out"=w275:refnum<class "XuLyDataDisplay.lvclass">)  [unwired: 7 in]
              }
              event "MAX ACCEL.Config_SetMaxACCEL": Value Change {
                n107 = event-data() -> ("NewVal"=w293:bool)  [unwired: 1 in]
                n108 = call "CheckButtoneTrue.vi"("IN"=w293) -> ("OUT"=w292:bool)  [unwired: 10 in]
                n109 = Unbundle By Name("MAX ACCEL") -> ("DATA"=w282:cluster{"X":dbl, "Y":dbl, "Z":dbl})
                n110 = To Variant(anything=w282) -> (Variant=w284:variant)
                n111 = call-dynamic "initMcode.vi"("CheckMenu"=w292, "error in (no error)"=w290, "mCode"=SelectMcode."M201_SetMaxACCEL", "DataVariant"=w284, "XuLyDataDisplay in"=w291) -> ("error out"=w287:errorcluster, "McodeOut"=w288:string, "XuLyDataDisplay out"=w289:refnum<class "XuLyDataDisplay.lvclass">)  [unwired: 4 in]
                n112 = call-dynamic "WriteDataToQueueCMD.vi"("error in (no error)"=w287, "DataIn"=w288, "ParameterConf in"=w289) -> ("error out"=w285:errorcluster, "ParameterConf out"=w286:refnum<class "XuLyDataDisplay.lvclass">)  [unwired: 7 in]
              }
              event "STEPSIZE.Config_SetStepSize": Value Change {
                n113 = event-data() -> ("NewVal"=w305:bool)  [unwired: 1 in]
                n114 = call "CheckButtoneTrue.vi"("IN"=w305) -> ("OUT"=w298:bool)  [unwired: 10 in]
                n115 = Unbundle By Name("STEPSIZE") -> ("DATA"=w296:cluster{"X":dbl, "Y":dbl, "Z":dbl})
                n116 = To Variant(anything=w296) -> (Variant=w297:variant)
                n117 = call-dynamic "initMcode.vi"("CheckMenu"=w298, "error in (no error)"=w299, "mCode"=SelectMcode."M92_SetAxisStepPerUnit", "DataVariant"=w297, "XuLyDataDisplay in"=w304) -> ("error out"=w300:errorcluster, "XuLyDataDisplay out"=w303:refnum<class "XuLyDataDisplay.lvclass">)  [unwired: 4 in, 1 out]
                n118 = call-dynamic "WriteDataToQueueCMD.vi"("error in (no error)"=w300, "ParameterConf in"=w303) -> ("error out"=w301:errorcluster, "ParameterConf out"=w302:refnum<class "XuLyDataDisplay.lvclass">)  [unwired: 8 in]
              }
              event "Config_SaveEEPROM": Value Change {
                n119 = event-data() -> ("NewVal"=w315:bool)  [unwired: 1 in]
                n120 = call "CheckButtoneTrue.vi"("IN"=w315) -> ("OUT"=w308:bool)  [unwired: 10 in]
                n121 = call-dynamic "initMcode.vi"("CheckMenu"=w308, "error in (no error)"=w313, "mCode"=SelectMcode."M500_SaveEprom", "XuLyDataDisplay in"=w314) -> ("error out"=w309:errorcluster, "McodeOut"=w307:string, "XuLyDataDisplay out"=w312:refnum<class "XuLyDataDisplay.lvclass">)  [unwired: 5 in]
                n122 = call-dynamic "WriteDataToQueueCMD.vi"("error in (no error)"=w309, "DataIn"=w307, "ParameterConf in"=w312) -> ("error out"=w310:errorcluster, "ParameterConf out"=w311:refnum<class "XuLyDataDisplay.lvclass">)  [unwired: 7 in]
              }
              event "Send Gcode manual.SEND GCODE": Value Change {
                n123 = event-data() -> ()  [unwired: 1 in, 1 out]
                n124 = Unbundle By Name("Send Gcode manual") -> ("GCODE USET INPUT"=w325:string)
                n125 = call-dynamic "initGcode.vi"("gCode"=SelectGcode."sendGcodeString", "error in (no error)"=w326, "Gcode In"=w325, "XuLyDataDisplay in"=w328) -> ("error out"=w323:errorcluster, "GcodeString Out"=w320:string, "XuLyDataDisplay out"=w324:refnum<class "XuLyDataDisplay.lvclass">)  [unwired: 5 in]
                n126 = call-dynamic "WriteDataToQueueCMD.vi"("error in (no error)"=w323, "DataIn"=w320, "ParameterConf in"=w324) -> ("error out"=w321:errorcluster, "ParameterConf out"=w322:refnum<class "XuLyDataDisplay.lvclass">)  [unwired: 7 in]
                n127 = call-dynamic "ReadEmptyString.vi"("XuLyDataDisplay in"=w322) -> ("Boolean"=w318:bool, "String"=w317:string, "XuLyDataDisplay out"=w319:refnum<class "XuLyDataDisplay.lvclass">)  [unwired: 7 in, 1 out]
                n128 = Bundle("String"=w317, "Boolean"=w318) -> (w316:cluster{"String":string, "Boolean":bool})  [unwired: 1 in]
                n129 = property on="Send Gcode manual" class="Clust"("Val(Sgnl)"=w316) -> ()  [unwired: 2 in, 2 out]
              }
              event "Start Auto": Value Change {
                n130 = event-data() -> ("NewVal"=w333:bool)  [unwired: 1 in]
                n131 = global write "StartAutoandGcode.vi" "Start Auto"(w333) -> ()
                n132 = call "GCode File to Array.vi"("File Path"="File to Cut") -> ("G-Code Array"=w330:string[])  [unwired: 10 in]
                "G-Code Array 2" <- w330
                n133 = global write "StartAutoandGcode.vi" "G-Code Array 2"(w330) -> ()
              }
              event "Move.OK Button": Value Change {
                w349 = 0.0 ("X0")
                n134 = event-data() -> ()  [unwired: 1 in, 6 out]
                n135 = call-dynamic "Read PARA.vi"("error in (no error)"=w344, "ParameterConf in"=w345) -> ("error out"=w337:errorcluster, "ParameterConf out"=w343:refnum<class "XuLyDataDisplay.lvclass">)  [unwired: 6 in, 2 out]
                n136 = Unbundle By Name("Move") -> ("X"=w354:dbl, "Y"=w353:dbl)
                n137 = call "ScaraInverseKinematics.vi"("Y0"=w349, "X0"=w349, "L3"=w349, "L2"=23.0, "L1"=43.0, "Y"=w353, "X"=w354) -> ("angle 2"=w348:dbl, "angle 1"=w346:dbl)  [unwired: 3 in]
                n138 = Add(x=w346, y=w348) -> (x+y=w347:dbl)
                n139 = Bundle("angle 1"=w346, w347, 0) -> (w338:cluster{"angle 1":dbl, dbl, i32})  [unwired: 1 in]
                "output cluster 2" <- w338
                n140 = call-dynamic "initGcode.vi"("gCode"=SelectGcode."G1XY", "error in (no error)"=w337, "PosSetG92"=w338, "XuLyDataDisplay in"=w343) -> ("error out"=w341:errorcluster, "GcodeString Out"=w340:string, "XuLyDataDisplay out"=w342:refnum<class "XuLyDataDisplay.lvclass">)  [unwired: 5 in]
                n141 = call-dynamic "WriteDataToQueueCMD.vi"("error in (no error)"=w341, "DataIn"=w340, "ParameterConf in"=w342) -> ("error out"=w336:errorcluster, "ParameterConf out"=w335:refnum<class "XuLyDataDisplay.lvclass">)  [unwired: 7 in]
              }
              event "CONTROL PWM.WAIT PIN.PIN INPUT", "CONTROL PWM.FAN 3.PWM", "CONTROL PWM.FAN 2.PWM", "CONTROL PWM.FAN 1.PWM", "CONTROL PWM.SPIN.PWM", "PARA": Value Change {
                n142 = event-data() -> ()  [unwired: 1 in, 6 out]
              }
              event "BUTTON CONTROL MANUAL.Control_ButtonX-": Value Change {
                n143 = event-data() -> ("NewVal"=w368:bool)  [unwired: 1 in]
                n144 = call "CheckButtoneTrue.vi"("IN"=w368) -> ("OUT"=w361:bool)  [unwired: 10 in]
                n145 = call-dynamic "initGcode.vi"("Che Do"=w361, "gCode"=SelectGcode."JogX-", "error in (no error)"=w363, "XuLyDataDisplay in"=w364) -> ("error out"=w366:errorcluster, "GcodeString Out"=w360:string, "XuLyDataDisplay out"=w367:refnum<class "XuLyDataDisplay.lvclass">)  [unwired: 5 in]
                n146 = call-dynamic "WriteDataToQueueCMD.vi"("error in (no error)"=w366, "DataIn"=w360, "ParameterConf in"=w367) -> ("error out"=w362:errorcluster, "ParameterConf out"=w359:refnum<class "XuLyDataDisplay.lvclass">)  [unwired: 7 in]
              }
              event "CONTROL PWM.SOLENOID.AddFile_ButtonSolenoid": Value Change {
                n147 = event-data() -> ("NewVal"=w384:bool)  [unwired: 1 in]
                n148 = call "CheckButtoneTrue.vi"("IN"=w384) -> ("OUT"=w374:bool)  [unwired: 10 in]
                n149 = call-dynamic "ReadParameter.vi"("ParameterConf in"=w383, "error in (no error)"=w382, "Parameter"=T23."Solenoid") -> ("ParameterConf out"=w381:refnum<class "XuLyDataDisplay.lvclass">, "DataOutClust"=w372:T26, "error out"=w379:errorcluster)  [unwired: 4 in, 1 out]
                n150 = Unbundle By Name(w372) -> ("PWM"=w371:dbl)
                n151 = To Variant(anything=w371) -> (Variant=w376:variant)
                n152 = call-dynamic "initMcode.vi"("CheckMenu"=w374, "error in (no error)"=w379, "mCode"=SelectMcode."M380_381_SetSoleNoid_On_Off", "DataVariant"=w376, "XuLyDataDisplay in"=w381) -> ("error out"=w378:errorcluster, "McodeOut"=w375:string, "XuLyDataDisplay out"=w380:refnum<class "XuLyDataDisplay.lvclass">)  [unwired: 4 in]
                n153 = call-dynamic "InsetStringToFileGcode.vi"("error in (no error)"=w378, "StringFileGcode"=w375, "ParameterConf in"=w380) -> ("error out"=w369:errorcluster, "ParameterConf out"=w370:refnum<class "XuLyDataDisplay.lvclass">)  [unwired: 7 in]
              }
              event "CONTROL PWM.FAN 3.AddFile_ButtonFan3": Value Change {
                n154 = event-data() -> ("NewVal"=w399:bool)  [unwired: 1 in]
                n155 = call "CheckButtoneTrue.vi"("IN"=w399) -> ("OUT"=w390:bool)  [unwired: 10 in]
                n156 = call-dynamic "ReadParameter.vi"("ParameterConf in"=w398, "error in (no error)"=w397, "Parameter"=T23."Fan3") -> ("ParameterConf out"=w396:refnum<class "XuLyDataDisplay.lvclass">, "DataOutClust"=w388:T26, "error out"=w395:errorcluster)  [unwired: 4 in, 1 out]
                n157 = Unbundle By Name(w388) -> ("PWM"=w387:dbl)
                n158 = call-dynamic "initMcode.vi"("CheckMenu"=w390, "error in (no error)"=w395, "mCode"=SelectMcode."M106_SetFan3", "DataVariant"=w387, "XuLyDataDisplay in"=w396) -> ("error out"=w393:errorcluster, "McodeOut"=w392:string, "XuLyDataDisplay out"=w394:refnum<class "XuLyDataDisplay.lvclass">)  [unwired: 4 in]
                n159 = call-dynamic "InsetStringToFileGcode.vi"("error in (no error)"=w393, "StringFileGcode"=w392, "ParameterConf in"=w394) -> ("error out"=w385:errorcluster, "ParameterConf out"=w386:refnum<class "XuLyDataDisplay.lvclass">)  [unwired: 7 in]
              }
              event "CONTROL PWM.FAN 2.AddFile_ButtonFan2": Value Change {
                n160 = event-data() -> ("NewVal"=w414:bool)  [unwired: 1 in]
                n161 = call-dynamic "ReadParameter.vi"("ParameterConf in"=w409, "error in (no error)"=w408, "Parameter"=T23."Fan2") -> ("ParameterConf out"=w413:refnum<class "XuLyDataDisplay.lvclass">, "DataOutClust"=w403:T26, "error out"=w412:errorcluster)  [unwired: 4 in, 1 out]
                n162 = call "CheckButtoneTrue.vi"("IN"=w414) -> ("OUT"=w405:bool)  [unwired: 10 in]
                n163 = Unbundle By Name(w403) -> ("PWM"=w402:dbl)
                n164 = call-dynamic "initMcode.vi"("CheckMenu"=w405, "error in (no error)"=w412, "mCode"=SelectMcode."M106_SetFan2", "DataVariant"=w402, "XuLyDataDisplay in"=w413) -> ("error out"=w410:errorcluster, "McodeOut"=w407:string, "XuLyDataDisplay out"=w411:refnum<class "XuLyDataDisplay.lvclass">)  [unwired: 4 in]
                n165 = call-dynamic "InsetStringToFileGcode.vi"("error in (no error)"=w410, "StringFileGcode"=w407, "ParameterConf in"=w411) -> ("error out"=w400:errorcluster, "ParameterConf out"=w401:refnum<class "XuLyDataDisplay.lvclass">)  [unwired: 7 in]
              }
              event "CONTROL PWM.FAN 1.AddFile_ButtonFan1": Value Change {
                n166 = event-data() -> ("NewVal"=w427:bool)  [unwired: 1 in]
                n167 = call-dynamic "Read FAN1.vi"("error in (no error)"=w425, "ParameterConf in"=w426) -> ("error out"=w423:errorcluster, "FAN1"=w419:dbl, "ParameterConf out"=w422:refnum<class "XuLyDataDisplay.lvclass">)  [unwired: 6 in, 1 out]
                n168 = call "CheckButtoneTrue.vi"("IN"=w427) -> ("OUT"=w417:bool)  [unwired: 10 in]
                n169 = call-dynamic "initMcode.vi"("CheckMenu"=w417, "error in (no error)"=w423, "mCode"=SelectMcode."M106_SetFan1", "DataVariant"=w419, "XuLyDataDisplay in"=w422) -> ("error out"=w424:errorcluster, "McodeOut"=w420:string, "XuLyDataDisplay out"=w421:refnum<class "XuLyDataDisplay.lvclass">)  [unwired: 4 in]
                n170 = call-dynamic "InsetStringToFileGcode.vi"("error in (no error)"=w424, "StringFileGcode"=w420, "ParameterConf in"=w421) -> ("error out"=w415:errorcluster, "ParameterConf out"=w416:refnum<class "XuLyDataDisplay.lvclass">)  [unwired: 7 in]
              }
              event "CONTROL PWM.SPIN.ButtonSPINDLE_ADD_FILE": Value Change {
                n171 = event-data() -> ("NewVal"=w442:bool)  [unwired: 1 in]
                n172 = call "CheckButtoneTrue.vi"("IN"=w442) -> ("OUT"=w433:bool)  [unwired: 10 in]
                n173 = call-dynamic "ReadParameter.vi"("ParameterConf in"=w441, "error in (no error)"=w440, "Parameter"=T23."Spindle") -> ("ParameterConf out"=w438:refnum<class "XuLyDataDisplay.lvclass">, "DataOutClust"=w431:T26, "error out"=w437:errorcluster)  [unwired: 4 in, 1 out]
                n174 = Unbundle By Name(w431) -> ("PWM"=w430:dbl)
                n175 = call-dynamic "initMcode.vi"("CheckMenu"=w433, "error in (no error)"=w437, "mCode"=SelectMcode."M3_SetSpindle", "DataVariant"=w430, "XuLyDataDisplay in"=w438) -> ("error out"=w436:errorcluster, "McodeOut"=w435:string, "XuLyDataDisplay out"=w439:refnum<class "XuLyDataDisplay.lvclass">)  [unwired: 4 in]
                n176 = call-dynamic "InsetStringToFileGcode.vi"("error in (no error)"=w436, "StringFileGcode"=w435, "ParameterConf in"=w439) -> ("error out"=w428:errorcluster, "ParameterConf out"=w429:refnum<class "XuLyDataDisplay.lvclass">)  [unwired: 7 in]
              }
              event "BUTTON CONTROL GCODE FILE.FILE.AddFile_ButtonDeleteLastLine": Value Change {
                n177 = event-data() -> ("NewVal"=w448:bool)  [unwired: 1 in]
                n178 = call "CheckButtoneTrue.vi"("IN"=w448) -> ("OUT"=w445:bool)  [unwired: 10 in]
                n179 = call-dynamic "deleteLastLine.vi"("TypeControl"=w445, "error in (no error)"=w446, "XuLyDataDisplay in"=w447) -> ("error out"=w443:errorcluster, "XuLyDataDisplay out"=w444:refnum<class "XuLyDataDisplay.lvclass">)  [unwired: 7 in]
              }
              event "CONTROL PWM.WAIT PIN.Control_ButtonWaitPin": Value Change {
                n180 = event-data() -> ()  [unwired: 1 in, 1 out]
              }
              event "BUTTON CONTROL GCODE FILE.FILE.AddFile_ButtonDeleteAll": Value Change {
                n181 = event-data() -> ()  [unwired: 1 in, 1 out]
                n182 = call-dynamic "Write StringFileGcode.vi"("error in (no error)"=w452, "StringFileGcode"="", "ParameterConf in"=w455) -> ("error out"=w453:errorcluster, "ParameterConf out"=w451:refnum<class "XuLyDataDisplay.lvclass">)  [unwired: 7 in]
              }
              event "BUTTON CONTROL GCODE FILE.MOTION.AddFile_ButtonGoHome": Value Change {
                n183 = event-data() -> ("NewVal"=w465:bool)  [unwired: 1 in]
                n184 = call "CheckButtoneTrue.vi"("IN"=w465) -> ("OUT"=w458:bool)  [unwired: 10 in]
                n185 = call-dynamic "initGcode.vi"("Che Do"=w458, "gCode"=SelectGcode."G28AutoHome", "error in (no error)"=w461, "XuLyDataDisplay in"=w463) -> ("error out"=w460:errorcluster, "GcodeString Out"=w457:string, "XuLyDataDisplay out"=w462:refnum<class "XuLyDataDisplay.lvclass">)  [unwired: 5 in]
                n186 = call-dynamic "InsetStringToFileGcode.vi"("error in (no error)"=w460, "StringFileGcode"=w457, "ParameterConf in"=w462) -> ("error out"=w464:errorcluster, "ParameterConf out"=w456:refnum<class "XuLyDataDisplay.lvclass">)  [unwired: 7 in]
              }
              event "BUTTON CONTROL GCODE FILE.FILE.AddFile_ButtonSaveFile": Value Change {
                n187 = event-data() -> ("NewVal"=w475:bool)  [unwired: 1 in]
                n188 = call "CheckButtoneTrue.vi"("IN"=w475) -> ("OUT"=w466:bool)  [unwired: 10 in]
                n189 = call-dynamic "Read StringFileGcode.vi"("error in (no error)"=w473, "ParameterConf in"=w474) -> ("error out"=w469:errorcluster, "StringFileGcode"=w471:string, "ParameterConf out"=w472:refnum<class "XuLyDataDisplay.lvclass">)  [unwired: 7 in]
                n190 = call-dynamic "SaveFile.vi"("TyprControl"=w466, "error in (no error)"=w469, "text"=w471, "file path (use dialog)"="Link Save File", "XuLyDataDisplay in"=w472) -> ("error out"=w467:errorcluster, "XuLyDataDisplay out"=w468:refnum<class "XuLyDataDisplay.lvclass">)  [unwired: 5 in]
              }
              event "BUTTON CONTROL GCODE FILE.MOTION.AddFile_ButtonAddG1": Value Change {
                n191 = event-data() -> ("NewVal"=w487:bool)  [unwired: 1 in]
                n192 = call-dynamic "Read PARA.vi"("error in (no error)"=w483, "ParameterConf in"=w486) -> ("error out"=w480:errorcluster, "ParameterConf out"=w482:refnum<class "XuLyDataDisplay.lvclass">)  [unwired: 6 in, 2 out]
                n193 = call "CheckButtoneTrue.vi"("IN"=w487) -> ("OUT"=w478:bool)  [unwired: 10 in]
                n194 = call-dynamic "initGcode.vi"("Che Do"=w478, "gCode"=SelectGcode."G1LinearMove", "error in (no error)"=w480, "XuLyDataDisplay in"=w482) -> ("error out"=w479:errorcluster, "GcodeString Out"=w476:string, "XuLyDataDisplay out"=w481:refnum<class "XuLyDataDisplay.lvclass">)  [unwired: 5 in]
                n195 = call-dynamic "InsetStringToFileGcode.vi"("error in (no error)"=w479, "StringFileGcode"=w476, "ParameterConf in"=w481) -> ("error out"=w484:errorcluster, "ParameterConf out"=w485:refnum<class "XuLyDataDisplay.lvclass">)  [unwired: 7 in]
              }
              event "BUTTON CONTROL GCODE FILE.MOTION.AddFile_ButtonAddG0": Value Change {
                n196 = event-data() -> ("NewVal"=w497:bool)  [unwired: 1 in]
                n197 = call "CheckButtoneTrue.vi"("IN"=w497) -> ("OUT"=w490:bool)  [unwired: 10 in]
                n198 = call-dynamic "initGcode.vi"("Che Do"=w490, "gCode"=SelectGcode."G0LinearMove", "error in (no error)"=w495, "XuLyDataDisplay in"=w496) -> ("error out"=w491:errorcluster, "GcodeString Out"=w488:string, "XuLyDataDisplay out"=w492:refnum<class "XuLyDataDisplay.lvclass">)  [unwired: 5 in]
                n199 = call-dynamic "InsetStringToFileGcode.vi"("error in (no error)"=w491, "StringFileGcode"=w488, "ParameterConf in"=w492) -> ("error out"=w493:errorcluster, "ParameterConf out"=w494:refnum<class "XuLyDataDisplay.lvclass">)  [unwired: 7 in]
              }
              event "BUTTON CONTROL MANUAL.Control_ButtonZ+": Value Change {
                n200 = event-data() -> ("NewVal"=w508:bool)  [unwired: 1 in]
                n201 = call "CheckButtoneTrue.vi"("IN"=w508) -> ("OUT"=w505:bool)  [unwired: 10 in]
                n202 = call-dynamic "initGcode.vi"("Che Do"=w505, "gCode"=SelectGcode."JogZ+", "error in (no error)"=w506, "XuLyDataDisplay in"=w507) -> ("error out"=w501:errorcluster, "GcodeString Out"=w499:string, "XuLyDataDisplay out"=w504:refnum<class "XuLyDataDisplay.lvclass">)  [unwired: 5 in]
                n203 = call-dynamic "WriteDataToQueueCMD.vi"("error in (no error)"=w501, "DataIn"=w499, "ParameterConf in"=w504) -> ("error out"=w502:errorcluster, "ParameterConf out"=w503:refnum<class "XuLyDataDisplay.lvclass">)  [unwired: 7 in]
              }
              event "BUTTON CONTROL MANUAL.Control_ButtonY+": Value Change {
                n204 = event-data() -> ("NewVal"=w518:bool)  [unwired: 1 in]
                n205 = call "CheckButtoneTrue.vi"("IN"=w518) -> ("OUT"=w515:bool)  [unwired: 10 in]
                n206 = call-dynamic "initGcode.vi"("Che Do"=w515, "gCode"=SelectGcode."JogY+", "error in (no error)"=w516, "XuLyDataDisplay in"=w517) -> ("error out"=w512:errorcluster, "GcodeString Out"=w513:string, "XuLyDataDisplay out"=w514:refnum<class "XuLyDataDisplay.lvclass">)  [unwired: 5 in]
                n207 = call-dynamic "WriteDataToQueueCMD.vi"("error in (no error)"=w512, "DataIn"=w513, "ParameterConf in"=w514) -> ("error out"=w509:errorcluster, "ParameterConf out"=w510:refnum<class "XuLyDataDisplay.lvclass">)  [unwired: 7 in]
              }
              event "BUTTON CONTROL MANUAL.Control_ButtonY-": Value Change {
                n208 = event-data() -> ("NewVal"=w528:bool)  [unwired: 1 in]
                n209 = call "CheckButtoneTrue.vi"("IN"=w528) -> ("OUT"=w521:bool)  [unwired: 10 in]
                n210 = call-dynamic "initGcode.vi"("Che Do"=w521, "gCode"=SelectGcode."JogY-", "error in (no error)"=w522, "XuLyDataDisplay in"=w523) -> ("error out"=w525:errorcluster, "GcodeString Out"=w526:string, "XuLyDataDisplay out"=w527:refnum<class "XuLyDataDisplay.lvclass">)  [unwired: 5 in]
                n211 = call-dynamic "WriteDataToQueueCMD.vi"("error in (no error)"=w525, "DataIn"=w526, "ParameterConf in"=w527) -> ("error out"=w519:errorcluster, "ParameterConf out"=w520:refnum<class "XuLyDataDisplay.lvclass">)  [unwired: 7 in]
              }
              event "BUTTON CONTROL MANUAL.Control_ButtonZ-": Value Change {
                n212 = event-data() -> ("NewVal"=w538:bool)  [unwired: 1 in]
                n213 = call "CheckButtoneTrue.vi"("IN"=w538) -> ("OUT"=w530:bool)  [unwired: 10 in]
                n214 = call-dynamic "initGcode.vi"("Che Do"=w530, "gCode"=SelectGcode."JogZ-", "error in (no error)"=w532, "XuLyDataDisplay in"=w533) -> ("error out"=w535:errorcluster, "GcodeString Out"=w536:string, "XuLyDataDisplay out"=w537:refnum<class "XuLyDataDisplay.lvclass">)  [unwired: 5 in]
                n215 = call-dynamic "WriteDataToQueueCMD.vi"("error in (no error)"=w535, "DataIn"=w536, "ParameterConf in"=w537) -> ("error out"=w531:errorcluster, "ParameterConf out"=w529:refnum<class "XuLyDataDisplay.lvclass">)  [unwired: 7 in]
              }
            }
          }
          frame "End" {
          }
          frame "writeGlobal" {
            n216 = Unbundle By Name("CONTROL PWM") -> ("SPIN.PWM"=w561:dbl, "FAN 2.PWM"=w560:dbl, "FAN 1.PWM"=w559:dbl, "FAN 3.PWM"=w558:dbl, "WAIT PIN.PIN INPUT"=w557:dbl, "SOLENOID.Control_ButtonSolenoid"=w556:bool)
            n217 = Unbundle By Name("PARA") -> ("STEP"=w548:i16, "FEEDRATE"=w547:dbl)
            n218 = Bundle By Name(cluster=cluster{"STEP":i16, "FEEDRATE":dbl} {"STEP"=0, "FEEDRATE"=0.0} ("PARA"), "STEP"=w548, "FEEDRATE"=w547) -> (w545:cluster{"STEP":i16, "FEEDRATE":dbl})
            n219 = Bundle By Name(cluster=T25 {"SPIN"=0.0, "FAN2"=0.0, "FAN1"=0.0, "FAN3"=0.0, "WAIT PIN "=0.0} ("CONTROL PWM"), "SPIN"=w561, "FAN2"=w560, "FAN1"=w559, "FAN3"=w558, "WAIT PIN"=w557) -> (w564:T25)
            n220 = call-dynamic "Updatevalue.vi"("ParameterConf in"=w555, "CONTROL PWM"=w564, "PARA"=w545, "error in (no error)"=w554) -> ("ParameterConf out"=w563:refnum<class "XuLyDataDisplay.lvclass">, "error out"=w562:errorcluster)  [unwired: 5 in]
            n221 = call-dynamic "UpdateSoleNoid.vi"("error in (no error)"=w562, "Boolean"=w556, "ParameterConf in"=w563) -> ("error out"=w552:errorcluster, "ParameterConf out"=w553:refnum<class "XuLyDataDisplay.lvclass">)  [unwired: 7 in]
          }
          frame "schedules500ms" {
            n222 = global read "StartAutoandGcode.vi" "StateModeSoftWare"() -> (→"statusMode":T2)
            n223 = call-dynamic "Read StringFileGcode.vi"("error in (no error)"=w571, "ParameterConf in"=w572) -> ("error out"=w568:errorcluster, "StringFileGcode"=→"GCODE ADD":string, "ParameterConf out"=w569:refnum<class "XuLyDataDisplay.lvclass">)  [unwired: 7 in]
          }
        }
        n224 = node-c288() -> ()  [unwired: 1 in, 1 out]
        n225 = call-dynamic "Write StateDisplay.vi"("error in (no error)"=w47, "StateDisplay"=w45, "ParameterConf in"=w44) -> ("error out"=w48:errorcluster, "ParameterConf out"=w49:refnum<class "XuLyDataDisplay.lvclass">)  [unwired: 7 in]
      }
      n226 = node-c288(w38) -> ()  [unwired: 1 out]
    }
  }
  n227 = Obtain Queue(name (unnamed)=w23, element data type=w23) -> (queue out=w19:refnum<queue>, error out=w7:errorcluster)  [unwired: 3 in, 1 out]
  n228 = Obtain Queue(element data type=T15 {"Command"=enum."updatePos", "POS"={"X"=0.0, "Y"=0.0, "Z"=0.0}, "DEGREES"={"X"=0.0, "Y"=0.0}}, error in (no error)=w7) -> (queue out=w8:refnum<queue>, error out=w17:errorcluster)  [unwired: 3 in, 1 out]
  n229 = Merge Errors(w17, w21, w22) -> (w13:errorcluster)
  n230 = Bundle(cluster=T16 {"Serial Data Gcode"=refnum, "cmdUpdateDisplay"=refnum}, "Serial Data Gcode"=w19, "cmdUpdateDisplay"=w8) -> (w14:T16)
  n231 = Bundle("cluster"=w14, "error IO"=w13) -> (w11:cluster{"cluster":T16, "error IO":errorcluster})  [unwired: 1 in]
  n232 = Unbundle By Name(w11) -> ("cluster"=w12:T16, "error IO"=w5:errorcluster)
  n233 = call "mainControlSerial.vi"("error in (no error)"=w5, "Queue In"=w12) -> ("error out"=w6:errorcluster)  [unwired: 9 in]
  n234 = call "mainControlAuto.vi"("error IO"=w5, "QueueCluste"=w12) -> ("error IO 2"=w16:errorcluster)  [unwired: 9 in]
  n235 = while {
    tunnel: w11 -> [_]
    shift-right: [w576] -> _
    shift-left: w9 -> [w582]
    shift-right: [w578] -> _
    shift-left: Robot_testing_instructions."Init 1 - Application" -> [w579]
    stop <- w580 stop-if-true
    n236 = case shown="\"Draw Robot\"" w579 {
      selector: w579 -> [_ _ _ w608 w611 w613 _]
      tunnel: w582 -> [w584 w585 w600 w609 w610 w612 w628]
      tunnel: [w584 w588 w599 w609 w610 w612 w627] -> w576
      tunnel: [Robot_testing_instructions."Error Handling" Robot_testing_instructions."Calculates" Robot_testing_instructions."Draw Robot" w608 w611 w613 Robot_testing_instructions."Calculates"] -> w578
      frame "idle", Default {
      }
      frame "Draw Robot" {
        n237 = Unbundle By Name(w585) -> ("Robot Definition"=w596:T12)
        n238 = call "Create Robot State Machine.vi"("Robot Definition"=w596) -> ("error out"=→"error out 2":errorcluster, "Cluster"=w595:T27)  [unwired: 9 in]
        n239 = Unbundle By Name(w595) -> ("Scene ref"=w589:refnum<vi>, "Sand box ref"=w590:refnum<vi>, "Arm 1 ref"=w591:refnum<vi>, "Arm 1 Offset"=w592:cluster{"X":sgl, "Y":sgl, "Z":sgl}[], "Arm 2 ref"=w593:refnum<vi>, "Arm 2 Offset"=w594:cluster{"X":sgl, "Y":sgl, "Z":sgl}[])
        n240 = Bundle By Name(cluster=w585, "Scene ref"=w589, "sand box"=w590, "Arm 1 ref"=w591, "Arm 1 offset"=w592, "Arm 2 ref"=w593, "Arm 2 offset"=w594) -> (w588:T13)
      }
      frame "Init 1 - Application" {
        n241 = Bundle By Name(cluster=w600, "Robot Definition.Base"=sgl 4.0, "Robot Definition.L1"=sgl 4.3, "Robot Definition.L2"=sgl 2.3, "Robot Definition.L3"=sgl 0.0, "Robot Definition.X0"=sgl 0.0, "Robot Definition.Z0"=sgl 0.0, "A1"=0.0, "A2"=0.0) -> (w599:T13)
      }
      frame "Quit" {
      }
      frame "Close" {
      }
      frame "Error Handling" {
      }
      frame "Calculates" {
        n242 = Unbundle By Name(w628) -> ("Arm 2 offset"=w642:cluster{"X":sgl, "Y":sgl, "Z":sgl}[], "Arm 2 ref"=w632:refnum<vi>, "Arm 1 offset"=w639:cluster{"X":sgl, "Y":sgl, "Z":sgl}[], "Arm 1 ref"=w636:refnum<vi>)
        n243 = local read "degrees"() -> (w617:cluster{"A":dbl, "B":dbl})
        n244 = Index Array(array=w639) -> (element #1=w635:cluster{"X":sgl, "Y":sgl, "Z":sgl}, element #2=w633:cluster{"X":sgl, "Y":sgl, "Z":sgl})  [unwired: 2 in]
        n245 = call <vilib>:"Clear Transformation.vi"("Object Refnum In"=w636) -> ("error out"=w626:errorcluster, "Object Refnum Out"=w641:refnum<vi>)  [unwired: 9 in]
        n246 = call <vilib>:"Set Translation.vi"("error in (no error)"=w626, "Translation"=w635, "Scene Object"=w641) -> ("error out"=w625:errorcluster, "Translated Object"=w637:refnum<vi>)  [unwired: 7 in]
        n247 = Unbundle By Name(w617) -> ("A"=w615:dbl, "B"=w616:dbl)
        n248 = call <vilib>:"Rotate Y-axis.vi"("Relative?"=TRUE, "error in (no error)"=w625, "angle"=w615, "Scene Object In"=w637) -> ("error out"=w624:errorcluster, "Scene Object Out"=w640:refnum<vi>)  [unwired: 6 in]
        n249 = call <vilib>:"Translate Object.vi"("error in (no error)"=w624, "Translation"=w633, "Scene.Object In"=w640) -> ("error out"=w623:errorcluster, "Scene.Object Out"=w638:refnum<vi>)  [unwired: 7 in]
        n250 = Subtract(x=w616, y=w615) -> (x-y=w614:dbl)
        n251 = call <vilib>:"Clear Transformation.vi"("error in (no error)"=w623, "Object Refnum In"=w632) -> ("error out"=w622:errorcluster, "Object Refnum Out"=w645:refnum<vi>)  [unwired: 8 in]
        n252 = Index Array(array=w642) -> (element #1=w631:cluster{"X":sgl, "Y":sgl, "Z":sgl}, element #2=w629:cluster{"X":sgl, "Y":sgl, "Z":sgl})  [unwired: 2 in]
        n253 = call <vilib>:"Set Translation.vi"("error in (no error)"=w622, "Translation"=w631, "Scene Object"=w645) -> ("error out"=w621:errorcluster, "Translated Object"=w646:refnum<vi>)  [unwired: 7 in]
        n254 = call <vilib>:"Rotate Y-axis.vi"("Relative?"=TRUE, "error in (no error)"=w621, "angle"=w614, "Scene Object In"=w646) -> ("error out"=w620:errorcluster, "Scene Object Out"=w644:refnum<vi>)  [unwired: 6 in]
        n255 = call <vilib>:"Translate Object.vi"("error in (no error)"=w620, "Translation"=w629, "Scene.Object In"=w644) -> ("error out"=→"error out":errorcluster, "Scene.Object Out"=w643:refnum<vi>)  [unwired: 7 in]
        n256 = Bundle By Name(cluster=w628, "Arm 1 ref"=w638, "Arm 2 ref"=w643) -> (w627:T13)
      }
    }
    n257 = Wait (ms)(milliseconds to wait=u32 10) -> ()  [unwired: 1 out]
    n258 = global read "StartAutoandGcode.vi" "EMG"() -> (w580:bool)
    n259 = Unbundle By Name(w576) -> ("Scene ref"=→"3D Picture":refnum<vi>)
  }
  n260 = Bundle("error out"=w6, "error IO 2"=w16) -> (w15:T28)  [unwired: 1 in]
  n261 = call-dynamic "Release Queue.vi"("error in (no error)"=w3, "ParameterConf in"=w4) -> ("error out"=w2:errorcluster)  [unwired: 8 in, 1 out]
  n262 = Unregister For Events(event registration refnum=w1) -> ()  [unwired: 1 in, 1 out]
  n263 = Bundle(w15, "error out"=w2) -> ()  [unwired: 1 in, 1 out]
